vi "executeCommand.vi"(8 "error in (no error)":errorcluster, 9 "parameter":variant, 10 "monoCommand":T2, 11 "MonoCommunicator in":refnum<class "MonoCommunicator.lvclass">) -> (0 "error out":errorcluster, 3 "MonoCommunicator out":refnum<class "MonoCommunicator.lvclass">)   [LabVIEW 2016, in "MonoCommunicator.lvclass"]
uses:
  MonoCommunicator.lvclass
  Typedefs/MonoCommand.ctl
  Typedefs/GratingType.ctl
  Typedefs/SlitType.ctl
  Typedefs/wavelength.ctl
  Typedefs/slitWidth.ctl
  Typedefs/AckType.ctl
  Typedefs/slit.ctl
panel:
  in  "GratingType":T1=enum."Red"
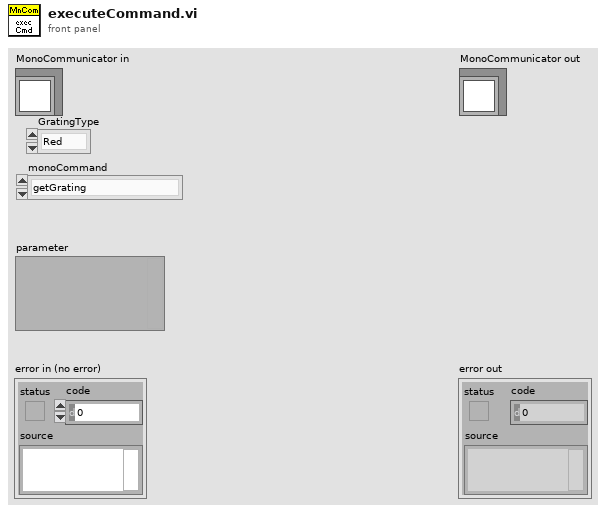
[diagram p1: front panel]
types:
  T1 = typedef "GratingType.ctl" = enum16{"Blue", "Red", "Mirror"}
  T2 = typedef "MonoCommand.ctl" = enum16{"getGrating", "getFrontEntranceSlitPosition", "getFrontExitSlitPosition", "getWavelength", "setWavelength", "setGrating", "setFrontEntranceSlitPosition", "setFrontExitSlitPosition", "calibrateWavelength", "getStatus", "Unknown", "reset"}
  T3 = typedef "SlitType.ctl" = enum16{"Front Entrance", "Side Entrance", "Front Exit", "Side Exit", "First Intermediate", "Second Intermediate"}
  T4 = typedef "slitWidth.ctl" = dbl
  T5 = typedef "wavelength.ctl" = dbl
  T6 = typedef "AckType.ctl" = enum16{"OK", "OutOfRange", "Unknown", "Busy", "Rejected"}
  T7 = typedef "slit.ctl" = cluster{"SlitType":T3, "Width":T4}
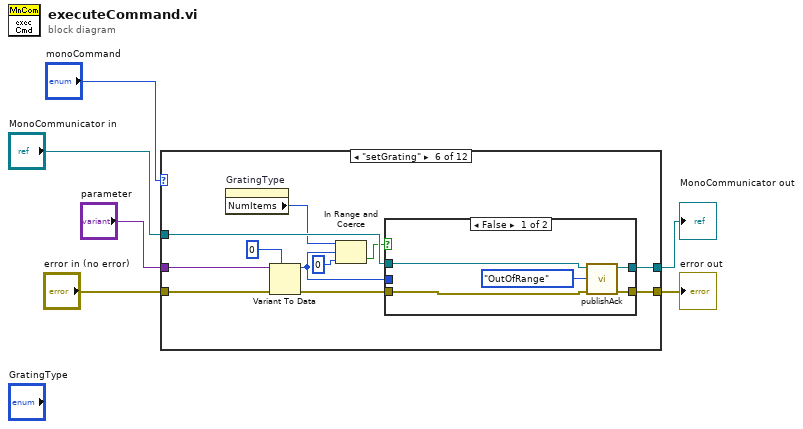
[diagram p0: block diagram]
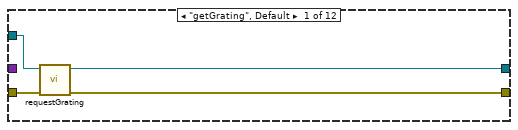
[diagram p2: hidden frame]
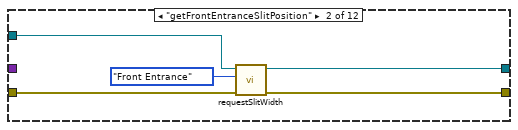
[diagram p3: hidden frame]
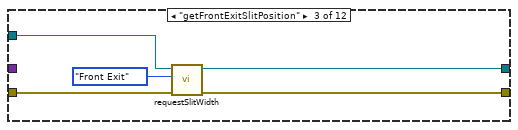
[diagram p4: hidden frame]
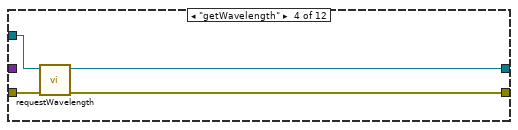
[diagram p5: hidden frame]
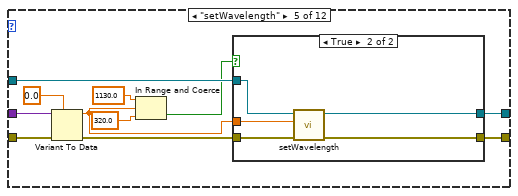
[diagram p6: hidden frame]
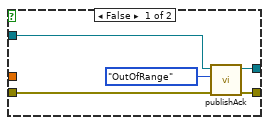
[diagram p7: hidden frame]
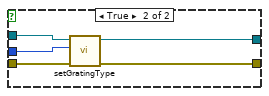
[diagram p8: hidden frame]
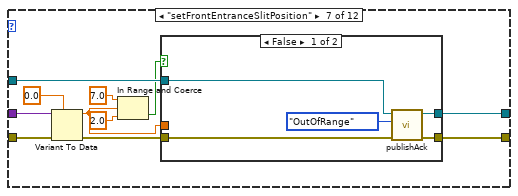
[diagram p9: hidden frame]
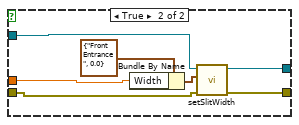
[diagram p10: hidden frame]
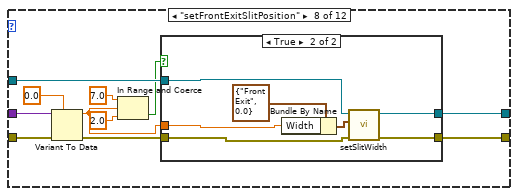
[diagram p11: hidden frame]
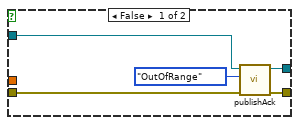
[diagram p12: hidden frame]
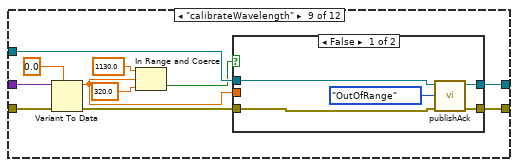
[diagram p13: hidden frame]
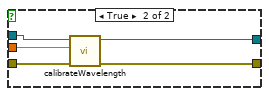
[diagram p14: hidden frame]
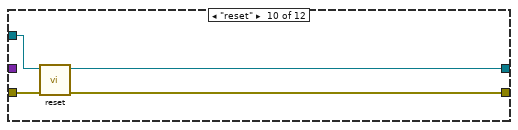
[diagram p15: hidden frame]
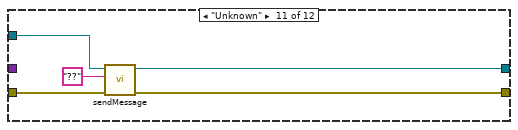
[diagram p16: hidden frame]
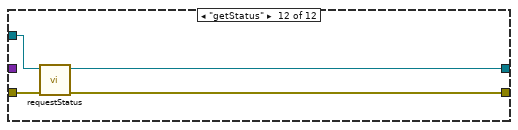
[diagram p17: hidden frame]
diagram:
  n1 = case shown="\"setGrating\"" "monoCommand" {
    tunnel: "MonoCommunicator in" -> [w7 w15 w20 w24 w35 w51 w75 w98 w123 w134 w142 w143]
    tunnel: [w8 w14 w19 w23 w34 w55 w76 w99 w122 w135 w141 w144] -> w4
    tunnel: "error in (no error)" -> [w10 w12 w17 w21 w32 w54 w71 w96 w120 w137 w140 w146]
    tunnel: [w9 w13 w18 w22 w33 w56 w77 w94 w121 w136 w139 w145] -> w2
    tunnel: "parameter" -> [_ _ _ _ w30 w52 w73 w97 w117 _ _ _]
    frame "getGrating", Default {
      n2 = call "requestGrating.vi"("error in (no error)"=w10, "MonoCommunicator in"=w7) -> ("error out"=w9:errorcluster, "MonoCommunicator out"=w8:refnum<class "MonoCommunicator.lvclass">)  [unwired: 8 in]
    }
    frame "getFrontEntranceSlitPosition" {
      n3 = call "requestSlitWidth.vi"("error in (no error)"=w12, "SlitType"=SlitType."Front Entrance", "MonoCommunicator in"=w15) -> ("error out"=w13:errorcluster, "MonoCommunicator out"=w14:refnum<class "MonoCommunicator.lvclass">)  [unwired: 7 in]
    }
    frame "getFrontExitSlitPosition" {
      n4 = call "requestSlitWidth.vi"("error in (no error)"=w17, "SlitType"=SlitType."Front Exit", "MonoCommunicator in"=w20) -> ("error out"=w18:errorcluster, "MonoCommunicator out"=w19:refnum<class "MonoCommunicator.lvclass">)  [unwired: 7 in]
    }
    frame "getWavelength" {
      n5 = call "requestWavelength.vi"("error in (no error)"=w21, "MonoCommunicator in"=w24) -> ("error out"=w22:errorcluster, "MonoCommunicator out"=w23:refnum<class "MonoCommunicator.lvclass">)  [unwired: 8 in]
    }
    frame "setWavelength" {
      n6 = Variant To Data(error in=w32, type=T5 0.0 ("wavelength"), Variant=w30) -> (data=w26:T5, error out=w31:errorcluster)
      n7 = In Range and Coerce(upper limit=T4 1130.0, x=w26, lower limit=T4 320.0) -> (In Range?=w25:bool)  [unwired: 1 out]
      n8 = case shown="True" w25 {
        tunnel: w35 -> [w38 w45]
        tunnel: [w37 w44] -> w34
        tunnel: [w36 w43] -> w33
        tunnel: w31 -> [w39 w42]
        tunnel: w26 -> [_ w41]
        frame False {
          n9 = call "publishAck.vi"("error in (no error)"=w39, "AckType"=AckType."OutOfRange", "MonoCommunicator in"=w38) -> ("error out"=w36:errorcluster, "MonoCommunicator out"=w37:refnum<class "MonoCommunicator.lvclass">)  [unwired: 7 in]
        }
        frame True {
          n10 = call "setWavelength.vi"("error in (no error)"=w42, "wavelength"=w41, "MonoCommunicator in"=w45) -> ("error out"=w43:errorcluster, "MonoCommunicator out"=w44:refnum<class "MonoCommunicator.lvclass">)  [unwired: 7 in]
        }
      }
    }
    frame "setGrating" {
      n11 = property on="GratingType" class="Enum (strict)"() -> ("NumItems"=w46:u32)  [unwired: 2 in, 2 out]
      n12 = Variant To Data(error in=w54, type=u16 0, Variant=w52) -> (data=w48:u16, error out=w53:errorcluster)
      n13 = In Range and Coerce(upper limit=w46, x=w48, lower limit=u32 0) -> (In Range?=w47:bool)  [unwired: 1 out]
      n14 = case shown="False" w47 {
        tunnel: [w59 w66] -> w56
        tunnel: [w58 w65] -> w55
        tunnel: w53 -> [w60 w64]
        tunnel: w48 -> [_ w63]
        tunnel: w51 -> [w57 w62]
        frame False {
          n15 = call "publishAck.vi"("error in (no error)"=w60, "AckType"=AckType."OutOfRange", "MonoCommunicator in"=w57) -> ("error out"=w59:errorcluster, "MonoCommunicator out"=w58:refnum<class "MonoCommunicator.lvclass">)  [unwired: 7 in]
        }
        frame True {
          n16 = call "setGratingType.vi"("error in (no error)"=w64, "GratingType"=w63, "MonoCommunicator in"=w62) -> ("error out"=w66:errorcluster, "MonoCommunicator out"=w65:refnum<class "MonoCommunicator.lvclass">)  [unwired: 7 in]
        }
      }
    }
    frame "setFrontEntranceSlitPosition" {
      n17 = Variant To Data(error in=w71, type=T4 0.0 ("position"), Variant=w73) -> (data=w69:T4, error out=w72:errorcluster)
      n18 = In Range and Coerce(upper limit=T4 7.0, x=w69, lower limit=T4 2.0) -> (In Range?=w70:bool)  [unwired: 1 out]
      n19 = case shown="False" w70 {
        tunnel: [w81 w89] -> w77
        tunnel: [w80 w88] -> w76
        tunnel: w75 -> [w79 w87]
        tunnel: w72 -> [w82 w84]
        tunnel: w69 -> [_ w83]
        frame False {
          n20 = call "publishAck.vi"("error in (no error)"=w82, "AckType"=AckType."OutOfRange", "MonoCommunicator in"=w79) -> ("error out"=w81:errorcluster, "MonoCommunicator out"=w80:refnum<class "MonoCommunicator.lvclass">)  [unwired: 7 in]
        }
        frame True {
          n21 = Bundle By Name(cluster=T7 {"SlitType"=enum."Front Entrance", "Width"=0.0} ("position"), "Width"=w83) -> (w85:T7)
          n22 = call "setSlitWidth.vi"("error in (no error)"=w84, "position"=w85, "MonoCommunicator in"=w87) -> ("error out"=w89:errorcluster, "MonoCommunicator out"=w88:refnum<class "MonoCommunicator.lvclass">)  [unwired: 7 in]
        }
      }
    }
    frame "setFrontExitSlitPosition" {
      n23 = Variant To Data(error in=w96, type=T4 0.0 ("position"), Variant=w97) -> (data=w91:T4, error out=w95:errorcluster)
      n24 = In Range and Coerce(upper limit=T4 7.0, x=w91, lower limit=T4 2.0) -> (In Range?=w90:bool)  [unwired: 1 out]
      n25 = case shown="True" w90 {
        tunnel: w91 -> [_ w110]
        tunnel: [w102 w109] -> w99
        tunnel: w98 -> [w103 w108]
        tunnel: w95 -> [w104 w107]
        tunnel: [w101 w106] -> w94
        frame False {
          n26 = call "publishAck.vi"("error in (no error)"=w104, "AckType"=AckType."OutOfRange", "MonoCommunicator in"=w103) -> ("error out"=w101:errorcluster, "MonoCommunicator out"=w102:refnum<class "MonoCommunicator.lvclass">)  [unwired: 7 in]
        }
        frame True {
          n27 = Bundle By Name(cluster=T7 {"SlitType"=enum."Front Exit", "Width"=0.0} ("position"), "Width"=w110) -> (w111:T7)
          n28 = call "setSlitWidth.vi"("error in (no error)"=w107, "position"=w111, "MonoCommunicator in"=w108) -> ("error out"=w106:errorcluster, "MonoCommunicator out"=w109:refnum<class "MonoCommunicator.lvclass">)  [unwired: 7 in]
        }
      }
    }
    frame "calibrateWavelength" {
      n29 = Variant To Data(error in=w120, type=T5 0.0 ("wavelength"), Variant=w117) -> (data=w113:T5, error out=w119:errorcluster)
      n30 = In Range and Coerce(upper limit=T4 1130.0, x=w113, lower limit=T4 320.0) -> (In Range?=w114:bool)  [unwired: 1 out]
      n31 = case shown="False" w114 {
        tunnel: w123 -> [w126 w133]
        tunnel: [w125 w132] -> w122
        tunnel: [w124 w131] -> w121
        tunnel: w119 -> [w127 w130]
        tunnel: w113 -> [_ w129]
        frame False {
          n32 = call "publishAck.vi"("error in (no error)"=w127, "AckType"=AckType."OutOfRange", "MonoCommunicator in"=w126) -> ("error out"=w124:errorcluster, "MonoCommunicator out"=w125:refnum<class "MonoCommunicator.lvclass">)  [unwired: 7 in]
        }
        frame True {
          n33 = call "calibrateWavelength.vi"("error in (no error)"=w130, "wavelength"=w129, "MonoCommunicator in"=w133) -> ("error out"=w131:errorcluster, "MonoCommunicator out"=w132:refnum<class "MonoCommunicator.lvclass">)  [unwired: 7 in]
        }
      }
    }
    frame "reset" {
      n34 = call "reset.vi"("error in (no error)"=w137, "MonoCommunicator in"=w134) -> ("error out"=w136:errorcluster, "MonoCommunicator out"=w135:refnum<class "MonoCommunicator.lvclass">)  [unwired: 8 in]
    }
    frame "Unknown" {
      n35 = call "sendMessage.vi"("error in (no error)"=w140, "message"="??", "MonoCommunicator in"=w142) -> ("error out"=w139:errorcluster, "MonoCommunicator out"=w141:refnum<class "MonoCommunicator.lvclass">)  [unwired: 7 in]
    }
    frame "getStatus" {
      n36 = call "requestStatus.vi"("error in (no error)"=w146, "MonoCommunicator in"=w143) -> ("error out"=w145:errorcluster, "MonoCommunicator out"=w144:refnum<class "MonoCommunicator.lvclass">)  [unwired: 8 in]
    }
  }
  "error out" <- w2
  "MonoCommunicator out" <- w4
